vi "Set_JPG_Path.vi"() -> ()   [LabVIEW 2015]
panel:
  out "链接后路径":path
  in  "volt2v":dbl
  in  "volt1v3":dbl
  in  "测试板编号":i32
  in  "source_path":path
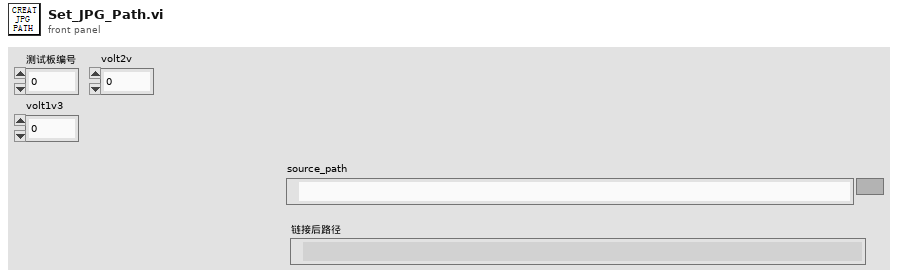
[diagram p1: front panel]
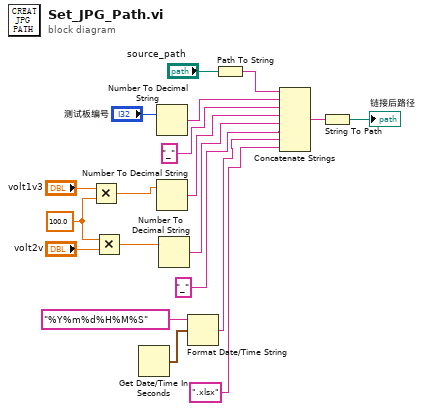
[diagram p0: block diagram]
diagram:
  w15 = 100.0
  n1 = Multiply(x="volt1v3", y=w15) -> (x*y=w12:dbl)
  n2 = Multiply(x=w15, y="volt2v") -> (x*y=w11:dbl)
  n3 = Get Date/Time In Seconds() -> (seconds since 1Jan1904=w6:timestamp)
  n4 = Number To Decimal String(number="测试板编号") -> (decimal integer string=w17:string)  [unwired: 1 in]
  n5 = Number To Decimal String(number=w12) -> (decimal integer string=w9:string)  [unwired: 1 in]
  n6 = Number To Decimal String(number=w11) -> (decimal integer string=w8:string)  [unwired: 1 in]
  n7 = Format Date/Time String(time format string (%c)="%Y%m%d%H%M%S" ("时间格式字符串(%c)"), seconds (now)=w6) -> (date/time string=w4:string)  [unwired: 1 in]
  n8 = Path To String(path="source_path") -> (string=w18:string)
  n9 = Concatenate Strings(w18, w17, "_", w9, w8, "_", w4, ".xlsx") -> (w2:string)
  n10 = String To Path(string=w2) -> (path=→"链接后路径":path)
